vi "运维调试_五参数.vi"(11 "编号":string) -> ()   [LabVIEW 2016, in "斯坦道多参数.lvlib"]
uses:
  <vilib>/Utility/miscctls.llb/LVPointTypeDef.ctl
  <vilib>/Plasmionique/MB Master/MB_Master_Serial/MB_Master_Serial.lvclass
  <vilib>/Utility/config.llb/NI_LVConfig.lvlib
panel:
  in  "权限2":bool
  out "权限1":bool
  out "密码":dbl
  in  "密码锁":bool
  in  "蓝绿藻探头选择":u16(ring) items=["禹山", "国弘", "纳清"]
  in  "叶绿素a探头选择":u16(ring) items=["禹山", "国弘", "纳清"]
  in  "浊度探头选择":u16(ring) items=["禹山", "国弘"]
  in  "电导率探头选择":u16(ring) items=["禹山", "国弘"]
  in  "DO探头选择":u16(ring) items=["禹山", "国弘"]
  in  "pH探头选择":u16(ring) items=["禹山", "国弘"]
  in  "设置页返回":bool
  in  "蓝绿藻":bool
  in  "打开串口":bool
  in  "叶绿素a启用":bool
  in  "Temp":bool
  in  "Cond":bool
  in  "Turb":bool
  in  "DO":bool
  in  "pH":bool
  in  "VISA资源名称":refnum<visa-resource-name>
  in  "周期设置":bool
  out "当前串口":string
  out "运行状态":u16(ring) items=["空闲", "水样测试", "标样核查"]
  in  "叶绿素a校准":bool
  in  "停止":bool
  in  "标样核查":bool
  in  "水样测试":bool
  in  "open MB":bool
  in  "设置":bool
  in  "水温校准":bool
  in  "浊度校准":bool
  in  "溶解氧校准":bool
  in  "电导率校准":bool
  in  "pH校准":bool
  in  "探头校正返回":bool
  in  "探头校正":bool
  out "检测值":T1
  # "请设置串口参数"
  # "请选择要启用的参数"
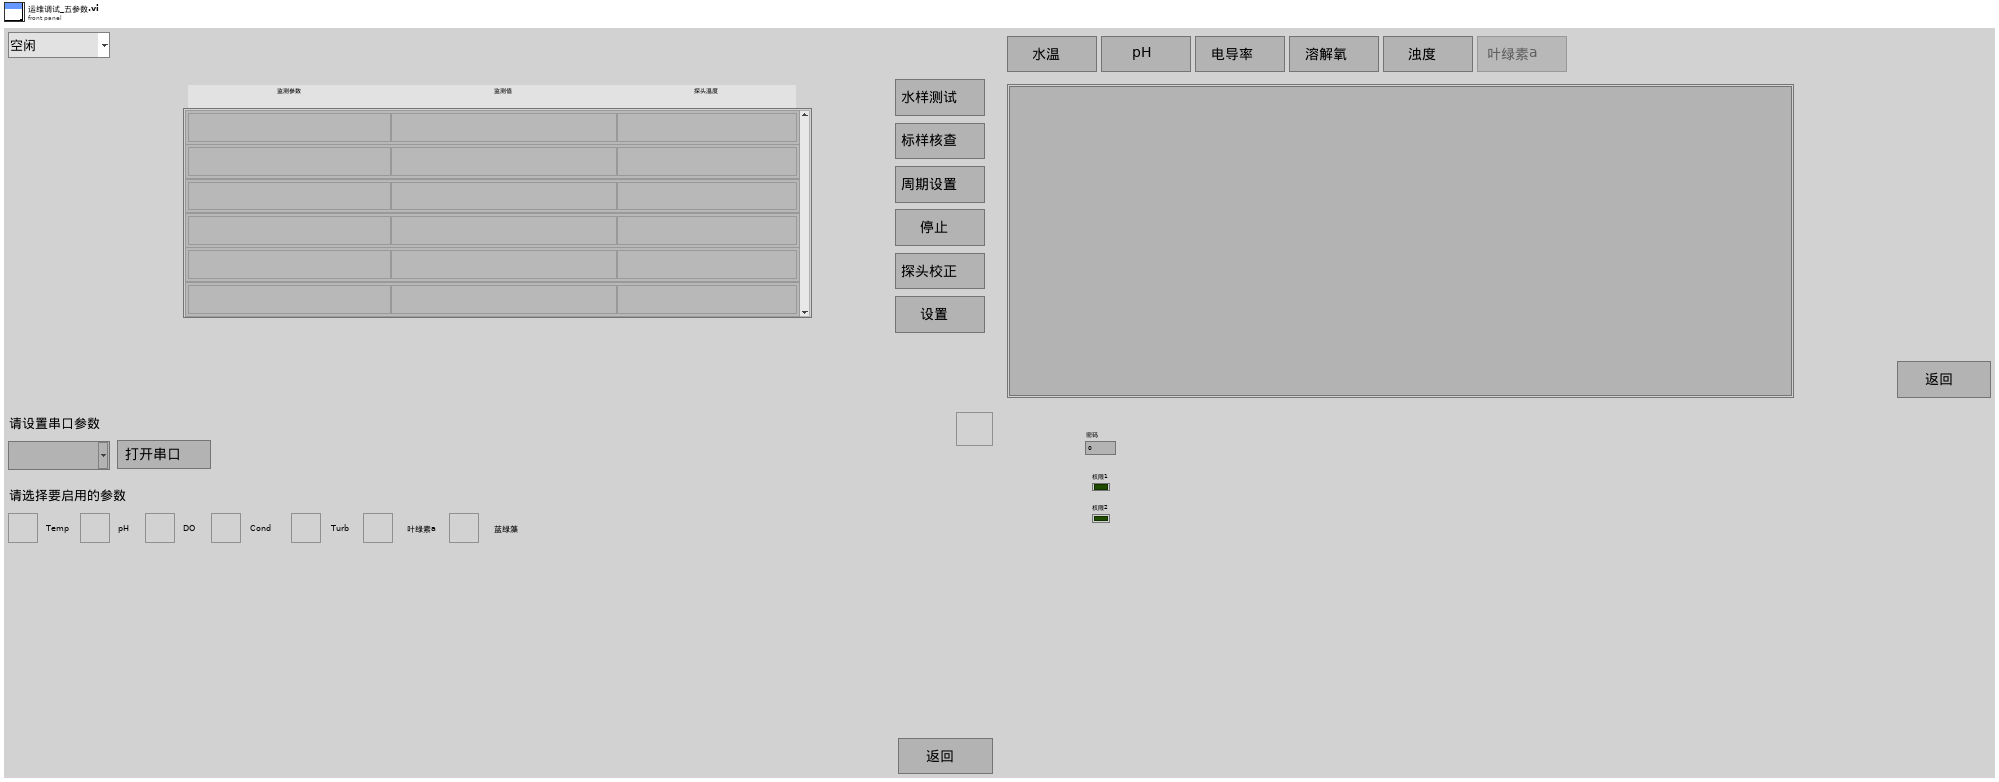
[diagram p1: front panel]
types:
  T1 = typedef "斯坦道多参数.lvlib/检测值.ctl" = cluster{"监测参数1":string, "浓度1":string, "探头温度1":string}[]
  T2 = typedef "LVPointTypeDef.ctl" = cluster{"Horizontal":i16, "Vertical":i16}
  T3 = cluster{"pH探头选择":u16, "DO探头选择":u16, "电导率探头选择":u16, "浊度探头选择":u16, "叶绿素a探头选择":u16, "蓝绿藻探头选择":u16}
  T4 = cluster{"温度测量值":sgl, "DO%":sgl, "DOmg/L":sgl, "温度偏移修正值":sgl}
  T5 = cluster{"电极状态标志":u16, "电极型号标志":u16, "溶解氧测量值":sgl, "温度测量值":sgl, "溶解氧饱和度值":sgl, "盐度补偿值":sgl, "大气压补偿值":sgl, "溶解氧偏移修正值":sgl, "温度偏移修正值":sgl, "手动温度补偿值":sgl, "溶解氧电极零点":sgl, "溶解氧电极斜率":sgl, "第1点标准值记录":sgl, "第1点信号值记录":sgl, "第1点温度值记录":sgl, "第2点标准值记录":sgl, "第2点信号值记录":sgl, "第2点温度值记录":sgl, "命令滤波设定":u16, "温度模式":enum16{"ATC", "MTC"}, "生产批次":u16, "电极序号":u16, "串口地址":u16, "串口波特率":enum16{"9600", "19200", "115200"}, "串口校验位":enum16{"NONE", "ODD", "EVEN"}, "串口停止位":enum16{"1bit", "2bit"}, "第一点标准值":sgl, "第二点标准值":sgl}
  T6 = cluster{"电极状态标志":u16, "电极型号标志":u16, "酸碱度测量值":sgl, "温度测量值":sgl, "酸碱度信号值":sgl, "温度信号值":sgl, "酸碱度偏移修正值":sgl, "温度偏移修正值":sgl, "手动温度补偿值":sgl, "酸碱度电极零点":sgl, "酸碱度电极斜率":sgl, "第1点标准值记录":sgl, "第1点信号值记录":sgl, "第1点温度值记录":sgl, "第2点标准值记录":sgl, "第2点信号值记录":sgl, "第2点温度值记录":sgl, "命令滤波设定":u16, "温度模式":enum16{"ATC", "MTC"}, "生产批次":u16, "电极序号":u16, "串口地址":u16, "串口波特率":enum16{"9600", "19200", "115200"}, "串口校验位":enum16{"NONE", "ODD", "EVEN"}, "串口停止位":enum16{"1bit", "2bit"}, "第一点标准值":sgl, "第二点标准值":sgl}
  T7 = cluster{"电极状态标志":u16, "电极型号标志":u16, "浊度测量值":sgl, "温度测量值":sgl, "浊度信号值":sgl, "浊度偏移修正值":sgl, "温度偏移修正值":sgl, "手动温度补偿值":sgl, "浊度电极零点":sgl, "浊度电极斜率":sgl, "第1点标准值记录":sgl, "第1点信号值记录":sgl, "第1点温度值记录":sgl, "第2点标准值记录":sgl, "第2点信号值记录":sgl, "第2点温度值记录":sgl, "命令滤波设定":u16, "温度模式":enum16{"ATC", "MTC"}, "生产批次":u16, "电极序号":u16, "串口地址":u16, "串口波特率":enum16{"9600", "19200", "115200"}, "串口校验位":enum16{"NONE", "ODD", "EVEN"}, "串口停止位":enum16{"1bit", "2bit"}, "第一点标准值":sgl, "第二点标准值":sgl, "第三点标准值":sgl}
  T8 = cluster{"电极状态标志":u16, "电极型号标志":u16, "电导率测量值":sgl, "温度测量值":sgl, "电导率信号值":sgl, "温度信号值":sgl, "温度补偿系数":sgl, "电导率偏移修正值":sgl, "温度偏移修正值":sgl, "手动温度补偿值":sgl, "电导率电极零点":sgl, "电导率电极斜率":sgl, "命令滤波设定":u16, "温度模式":enum16{"ATC", "MTC"}, "生产批次":u16, "电极序号":u16, "串口地址":u16, "串口波特率":enum16{"9600", "19200", "115200"}, "串口校验位":enum16{"NONE", "ODD", "EVEN"}, "串口停止位":enum16{"1bit", "2bit"}, "第一点标准值":sgl, "第二点标准值":sgl}
  T9 = enum8{"Enabled", "Disabled", "Disabled and Grayed Out"}
  T10 = cluster{"监测参数1":string, "浓度1":string, "探头温度1":string}[]
  T11 = cluster{"周期设置类型":enum16{"定点启动", "间隔启动"}, "定时功能启用":bool, "定时间隔":u32, "24H周期设置":bool[]}
  T12 = enum32{"Bad", "Idle", "Run top level", "Running"}
  T13 = typedef "LVDateTimeRec.ctl" = cluster{"秒数的小数部分":dbl, "秒":i32, "分":i32, "时":i32, "日":i32, "月":i32, "年":i32, "天数（周）":i32, "天数（年）":i32, "DST":i32}
  T14 = typedef "NI_LVConfig.lvlib/Config Data RefNum.ctl" = refnum<k1>
  T15 = cluster{"数据保存间隔":dbl, "水温标样值":dbl, "pH标样值":dbl, "溶解氧标样值":dbl, "电导率标样值":dbl, "浊度标样值":dbl}
  T16 = cluster{"baud rate (bps)":u32, "stop bits":u16, "parity":u16, "flow control":u16, "timeout":u32, "retries":i32}
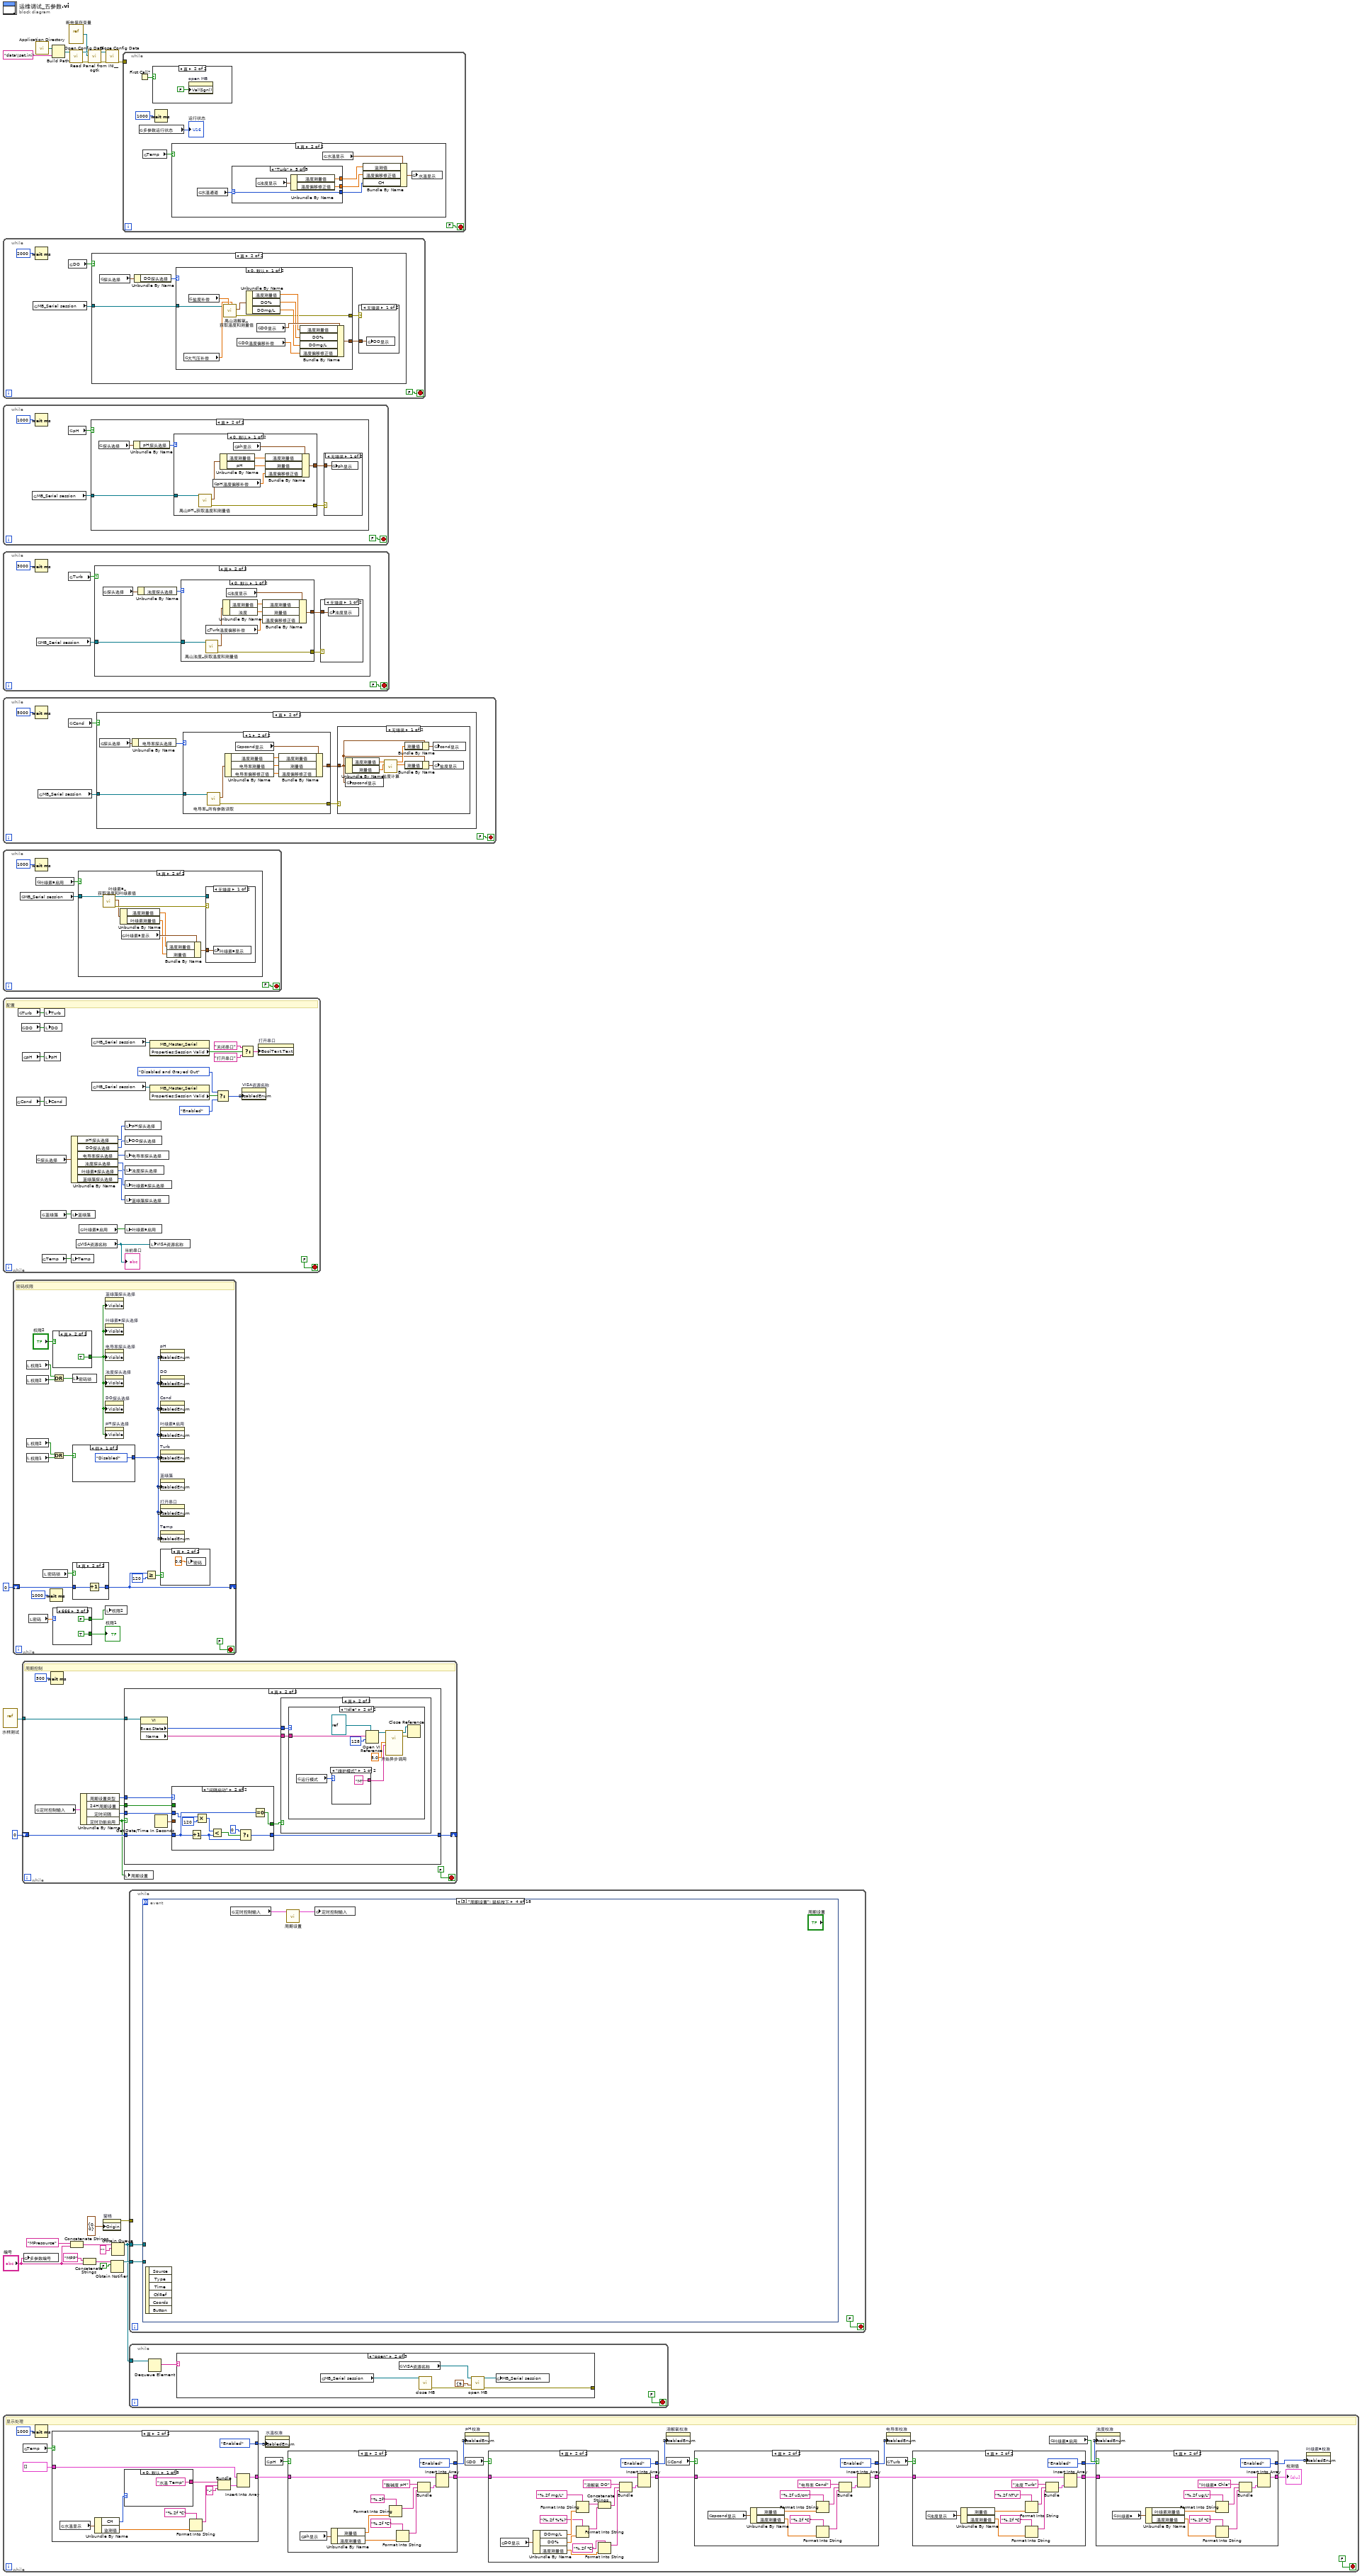
[diagram p0: block diagram]
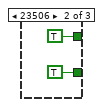
[diagram p5: hidden frame]
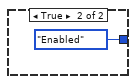
[diagram p6: hidden frame]
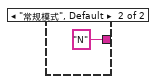
[diagram p11: hidden frame]
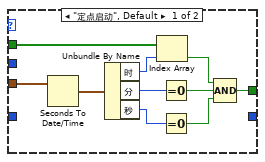
[diagram p12: hidden frame]
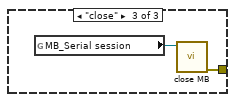
[diagram p14: hidden frame]
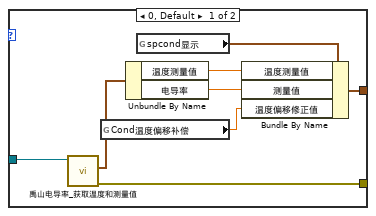
[diagram p18: hidden frame]
diagram:
  n1 = while {
    stop <- FALSE stop-if-true
    n2 = global read "多参数全局变量.vi" "MB_Serial session"() -> (w24:refnum<class "MB_Master_Serial.lvclass">)
    n3 = Wait (ms)(milliseconds to wait=u32 2000 ("等待时间（毫秒）")) -> ()  [unwired: 1 out]
    n4 = global read "断电保存变量.vi" "DO"() -> (w25:bool)
    n5 = case shown="真" w25 {
      tunnel: w24 -> [_ w30]
      frame False {
      }
      frame True {
        n6 = global read "断电保存变量.vi" "探头选择"() -> (w32:T3)
        n7 = Unbundle By Name(w32) -> ("DO探头选择"=w31:u16)
        n8 = case shown="0, 默认" w31 {
          tunnel: w30 -> [w41 w51]
          tunnel: [w39 w49] -> w29
          tunnel: [w35 w44] -> w28
          frame 0, Default {
            n9 = global read "断电保存变量.vi" "大气压补偿"() -> (w42:dbl)
            n10 = global read "断电保存变量.vi" "盐度补偿"() -> (w43:dbl)
            n11 = call "禹山溶解氧_获取温度和测量值.vi"("大气压补偿"=w42, "盐度补偿"=w43, "MB_Serial session in"=w41) -> ("error out"=w35:errorcluster, "输出值"=w33:cluster{"温度测量值":sgl, "DO%":sgl, "DOmg/L":sgl})  [unwired: 6 in, 1 out]
            n12 = global read "断电保存变量.vi" "DO温度偏移补偿"() -> (w34:dbl)
            n13 = Unbundle By Name(w33) -> ("温度测量值"=w38:sgl, "DO%"=w37:sgl, "DOmg/L"=w36:sgl)
            n14 = global read "多参数全局变量.vi" "DO显示"() -> (w40:T4)
            n15 = Bundle By Name(cluster=w40, "温度测量值"=w38, "DO%"=w37, "DOmg/L"=w36, "温度偏移修正值"=w34) -> (w39:T4)
          }
          frame 1 {
            n16 = call "DO_所有参数读取.vi"("MB_Serial session in"=w51) -> ("error out"=w44:errorcluster, "输出值"=w48:T5)  [unwired: 8 in, 1 out]
            n17 = Unbundle By Name(w48) -> ("温度测量值"=w45:sgl, "溶解氧饱和度值"=w46:sgl, "溶解氧测量值"=w47:sgl)
            n18 = global read "多参数全局变量.vi" "DO显示"() -> (w50:T4)
            n19 = Bundle By Name(cluster=w50, "温度测量值"=w45, "DO%"=w46, "DOmg/L"=w47) -> (w49:T4)
          }
        }
        n20 = case shown="无错误" w28 {
          tunnel: w29 -> [w52 _]
          frame No Error {
            n21 = global write "多参数全局变量.vi" "DO显示"(w52) -> ()
          }
          frame Error {
          }
        }
      }
    }
  }
  n22 = while {
    stop <- FALSE stop-if-true
    n23 = global read "多参数全局变量.vi" "MB_Serial session"() -> (w53:refnum<class "MB_Master_Serial.lvclass">)
    n24 = Wait (ms)(milliseconds to wait=u32 1000 ("等待时间（毫秒）")) -> ()  [unwired: 1 out]
    n25 = global read "断电保存变量.vi" "pH"() -> (w55:bool)
    n26 = case shown="真" w55 {
      tunnel: w53 -> [_ w59]
      frame False {
      }
      frame True {
        n27 = global read "断电保存变量.vi" "探头选择"() -> (w61:T3)
        n28 = Unbundle By Name(w61) -> ("pH探头选择"=w60:u16)
        n29 = case shown="0, 默认" w60 {
          tunnel: w59 -> [w69 w77]
          tunnel: [w68 w76] -> w58
          tunnel: [w66 w73] -> w57
          frame 0, Default {
            n30 = call "禹山pH_获取温度和测量值.vi"("MB_Serial session in"=w69) -> ("error out"=w68:errorcluster, "输出值"=w65:cluster{"温度测量值":sgl, "ORP":sgl, "pH":sgl})  [unwired: 8 in, 1 out]
            n31 = global read "断电保存变量.vi" "pH温度偏移补偿"() -> (w62:dbl)
            n32 = Unbundle By Name(w65) -> ("温度测量值"=w64:sgl, "pH"=w63:sgl)
            n33 = global read "多参数全局变量.vi" "ph显示"() -> (w67:cluster{"温度测量值":sgl, "测量值":sgl, "温度偏移修正值":sgl})
            n34 = Bundle By Name(cluster=w67, "温度测量值"=w64, "测量值"=w63, "温度偏移修正值"=w62) -> (w66:cluster{"温度测量值":sgl, "测量值":sgl, "温度偏移修正值":sgl})
          }
          frame 1 {
            n35 = call "pH_所有参数读取.vi"("MB_Serial session in"=w77) -> ("error out"=w76:errorcluster, "输出值"=w75:T6)  [unwired: 8 in, 1 out]
            n36 = Unbundle By Name(w75) -> ("温度测量值"=w70:sgl, "酸碱度测量值"=w71:sgl, "温度偏移修正值"=w72:sgl)
            n37 = global read "多参数全局变量.vi" "ph显示"() -> (w74:cluster{"温度测量值":sgl, "测量值":sgl, "温度偏移修正值":sgl})
            n38 = Bundle By Name(cluster=w74, "温度测量值"=w70, "测量值"=w71, "温度偏移修正值"=w72) -> (w73:cluster{"温度测量值":sgl, "测量值":sgl, "温度偏移修正值":sgl})
          }
        }
        n39 = case shown="无错误" w58 {
          tunnel: w57 -> [w78 _]
          frame No Error {
            n40 = global write "多参数全局变量.vi" "ph显示"(w78) -> ()
          }
          frame Error {
          }
        }
      }
    }
  }
  n41 = while {
    stop <- FALSE stop-if-true
    n42 = Wait (ms)(milliseconds to wait=u32 3000 ("等待时间（毫秒）")) -> ()  [unwired: 1 out]
    n43 = global read "多参数全局变量.vi" "MB_Serial session"() -> (w79:refnum<class "MB_Master_Serial.lvclass">)
    n44 = global read "断电保存变量.vi" "Turb"() -> (w81:bool)
    n45 = case shown="真" w81 {
      tunnel: w79 -> [_ w85]
      frame False {
      }
      frame True {
        n46 = global read "断电保存变量.vi" "探头选择"() -> (w87:T3)
        n47 = Unbundle By Name(w87) -> ("浊度探头选择"=w86:u16)
        n48 = case shown="0, 默认" w86 {
          tunnel: w85 -> [w95 w102]
          tunnel: [w93 w97] -> w84
          tunnel: [w92 w96] -> w83
          frame 0, Default {
            n49 = call "禹山浊度_获取温度和测量值.vi"("MB_Serial session in"=w95) -> ("error out"=w92:errorcluster, "输出值"=w91:cluster{"温度测量值":sgl, "浊度":sgl})  [unwired: 8 in, 1 out]
            n50 = global read "断电保存变量.vi" "Turb温度偏移补偿"() -> (w88:dbl)
            n51 = Unbundle By Name(w91) -> ("温度测量值"=w90:sgl, "浊度"=w89:sgl)
            n52 = global read "多参数全局变量.vi" "浊度显示"() -> (w94:cluster{"温度测量值":sgl, "测量值":sgl, "温度偏移修正值":sgl})
            n53 = Bundle By Name(cluster=w94, "温度测量值"=w90, "测量值"=w89, "温度偏移修正值"=w88) -> (w93:cluster{"温度测量值":sgl, "测量值":sgl, "温度偏移修正值":sgl})
          }
          frame 1 {
            n54 = call "浊度_所有参数读取.vi"("MB_Serial session in"=w102) -> ("error out"=w96:errorcluster, "输出值"=w101:T7)  [unwired: 8 in, 1 out]
            n55 = Unbundle By Name(w101) -> ("温度测量值"=w99:sgl, "浊度测量值"=w98:sgl)
            n56 = global read "多参数全局变量.vi" "浊度显示"() -> (w100:cluster{"温度测量值":sgl, "测量值":sgl, "温度偏移修正值":sgl})
            n57 = Bundle By Name(cluster=w100, "温度测量值"=w99, "测量值"=w98) -> (w97:cluster{"温度测量值":sgl, "测量值":sgl, "温度偏移修正值":sgl})
          }
        }
        n58 = case shown="无错误" w83 {
          tunnel: w84 -> [w103 _]
          frame No Error {
            n59 = global write "多参数全局变量.vi" "浊度显示"(w103) -> ()
          }
          frame Error {
          }
        }
      }
    }
  }
  n60 = while {
    stop <- FALSE stop-if-true
    n61 = Wait (ms)(milliseconds to wait=u32 5000 ("等待时间（毫秒）")) -> ()  [unwired: 1 out]
    n62 = global read "多参数全局变量.vi" "MB_Serial session"() -> (w104:refnum<class "MB_Master_Serial.lvclass">)
    n63 = global read "断电保存变量.vi" "Cond"() -> (w106:bool)
    n64 = case shown="真" w106 {
      tunnel: w104 -> [_ w110]
      frame False {
      }
      frame True {
        n65 = global read "断电保存变量.vi" "探头选择"() -> (w112:T3)
        n66 = Unbundle By Name(w112) -> ("电导率探头选择"=w111:u16)
        n67 = case shown="1" w111 {
          tunnel: w110 -> [w120 w128]
          tunnel: [w114 w126] -> w109
          tunnel: [w119 w125] -> w108
          frame 0, Default {
            n68 = call "禹山电导率_获取温度和测量值.vi"("MB_Serial session in"=w120) -> ("error out"=w119:errorcluster, "输出值"=w117:cluster{"温度测量值":sgl, "电导率":sgl, "错误标志":u16})  [unwired: 8 in, 1 out]
            n69 = global read "断电保存变量.vi" "Cond温度偏移补偿"() -> (w113:dbl)
            n70 = Unbundle By Name(w117) -> ("温度测量值"=w116:sgl, "电导率"=w115:sgl)
            n71 = global read "多参数全局变量.vi" "spcond显示"() -> (w118:cluster{"温度测量值":sgl, "测量值":sgl, "温度偏移修正值":sgl})
            n72 = Bundle By Name(cluster=w118, "温度测量值"=w116, "测量值"=w115, "温度偏移修正值"=w113) -> (w114:cluster{"温度测量值":sgl, "测量值":sgl, "温度偏移修正值":sgl})
          }
          frame 1 {
            n73 = call "电导率_所有参数读取.vi"("MB_Serial session in"=w128) -> ("error out"=w125:errorcluster, "输出值"=w124:T8)  [unwired: 8 in, 1 out]
            n74 = Unbundle By Name(w124) -> ("温度测量值"=w123:sgl, "电导率测量值"=w122:sgl, "电导率偏移修正值"=w121:sgl)
            n75 = global read "多参数全局变量.vi" "spcond显示"() -> (w127:cluster{"温度测量值":sgl, "测量值":sgl, "温度偏移修正值":sgl})
            n76 = Bundle By Name(cluster=w127, "温度测量值"=w123, "测量值"=w122, "温度偏移修正值"=w121) -> (w126:cluster{"温度测量值":sgl, "测量值":sgl, "温度偏移修正值":sgl})
          }
        }
        n77 = case shown="无错误" w108 {
          tunnel: w109 -> [w130 _]
          frame No Error {
            n78 = Unbundle By Name(w130) -> ("温度测量值"=w135:sgl, "测量值"=w134:sgl)
            n79 = global write "多参数全局变量.vi" "spcond显示"(w130) -> ()
            n80 = call "盐度计算.vi"("spCond"=w134, "Temp"=w135) -> ("saltresult"=w129:dbl, "cond"=w133:dbl)  [unwired: 8 in]
            n81 = Bundle By Name(cluster=w130, "测量值"=w133) -> (w132:cluster{"温度测量值":sgl, "测量值":sgl, "温度偏移修正值":sgl})
            n82 = Bundle By Name(cluster=w130, "测量值"=w129) -> (w131:cluster{"温度测量值":sgl, "测量值":sgl, "温度偏移修正值":sgl})
            n83 = global write "多参数全局变量.vi" "cond显示"(w132) -> ()
            n84 = global write "多参数全局变量.vi" "盐度显示"(w131) -> ()
          }
          frame Error {
          }
        }
      }
    }
  }
  n85 = while {
    stop <- FALSE stop-if-true
    n86 = global read "多参数全局变量.vi" "MB_Serial session"() -> (w136:refnum<class "MB_Master_Serial.lvclass">)
    n87 = Wait (ms)(milliseconds to wait=u32 1000 ("等待时间（毫秒）")) -> ()  [unwired: 1 out]
    n88 = global read "断电保存变量.vi" "叶绿素a启用"() -> (w138:bool)
    n89 = case shown="真" w138 {
      tunnel: w136 -> [_ w145]
      frame False {
      }
      frame True {
        n90 = call "叶绿素a_获取温度和叶绿素值.vi"("MB_Serial session in"=w145) -> ("error out"=w147:errorcluster, "输出值"=w142:cluster{"温度测量值":sgl, "叶绿素测量值":sgl, "错误标志":u16}, "MB_Serial session out"=w146:refnum<class "MB_Master_Serial.lvclass">)  [unwired: 8 in]
        n91 = Unbundle By Name(w142) -> ("温度测量值"=w140:sgl, "叶绿素测量值"=w141:sgl)
        n92 = global read "多参数全局变量.vi" "叶绿素a显示"() -> (w144:cluster{"温度测量值":sgl, "测量值":sgl, "温度偏移修正值":sgl})
        n93 = Bundle By Name(cluster=w144, "温度测量值"=w140, "测量值"=w141) -> (w143:cluster{"温度测量值":sgl, "测量值":sgl, "温度偏移修正值":sgl})
        n94 = case shown="无错误" w147 {
          tunnel: w146 -> [_ _]
          tunnel: w143 -> [w148 _]
          frame No Error {
            n95 = global write "多参数全局变量.vi" "叶绿素a显示"(w148) -> ()
          }
          frame Error {
          }
        }
      }
    }
  }
  n96 = while {
    stop <- FALSE stop-if-true
    # "配置"
    n97 = global read "断电保存变量.vi" "Cond"() -> (w170:bool)
    n98 = global read "断电保存变量.vi" "Turb"() -> (w169:bool)
    n99 = global read "断电保存变量.vi" "DO"() -> (w171:bool)
    n100 = global read "断电保存变量.vi" "pH"() -> (w172:bool)
    n101 = global read "断电保存变量.vi" "探头选择"() -> (w155:T3)
    n102 = global read "断电保存变量.vi" "蓝绿藻"() -> (w167:bool)
    n103 = global read "断电保存变量.vi" "Temp"() -> (w173:bool)
    n104 = local write "Turb"(w169) -> ()
    n105 = local write "DO"(w171) -> ()
    n106 = local write "pH"(w172) -> ()
    n107 = local write "Cond"(w170) -> ()
    n108 = Unbundle By Name(w155) -> ("pH探头选择"=w154:u16, "DO探头选择"=w153:u16, "电导率探头选择"=w152:u16, "浊度探头选择"=w151:u16, "叶绿素a探头选择"=w150:u16, "蓝绿藻探头选择"=w149:u16)
    n109 = local write "蓝绿藻"(w167) -> ()
    n110 = local write "Temp"(w173) -> ()
    n111 = global read "断电保存变量.vi" "VISA资源名称"() -> (w156:refnum<visa-resource-name>)
    "当前串口" <- w156
    n112 = global read "断电保存变量.vi" "叶绿素a启用"() -> (w168:bool)
    n113 = global read "多参数全局变量.vi" "MB_Serial session"() -> (w161:refnum<class "MB_Master_Serial.lvclass">)
    n114 = global read "多参数全局变量.vi" "MB_Serial session"() -> (w166:refnum<class "MB_Master_Serial.lvclass">)
    n115 = local write "pH探头选择"(w154) -> ()
    n116 = local write "DO探头选择"(w153) -> ()
    n117 = local write "电导率探头选择"(w152) -> ()
    n118 = local write "浊度探头选择"(w151) -> ()
    n119 = local write "叶绿素a探头选择"(w150) -> ()
    n120 = local write "蓝绿藻探头选择"(w149) -> ()
    n121 = local write "叶绿素a启用"(w168) -> ()
    n122 = property class="MB_Master_Serial"(reference=w161) -> ("Properties:Session Valid"=w160:bool)  [unwired: 1 in, 2 out]
    n123 = property class="MB_Master_Serial"(reference=w166) -> ("Properties:Session Valid"=w165:bool)  [unwired: 1 in, 2 out]
    n124 = local write "VISA资源名称"(w156) -> ()
    n125 = Select(t=T9."Disabled and Grayed Out" ("禁用"), s=w165, f=T9."Enabled") -> (s? t:f=w163:T9)
    n126 = Select(t="关闭串口" ("布尔文本.文本"), s=w160, f="打开串口" ("布尔文本.文本")) -> (s? t:f=w157:string)
    n127 = property on="VISA资源名称" class="VISAName"("DisabledEnum"=w163) -> ()  [unwired: 2 in, 2 out]
    n128 = property on="打开串口" class="Bool"("BoolText.Text"=w157) -> ()  [unwired: 2 in, 2 out]
  }
  n129 = vi-ref "水样测试.vi"() -> (w2:refnum<vi>)
  n130 = while {
    stop <- FALSE stop-if-true
    # "显示处理"
    n131 = global read "断电保存变量.vi" "Temp"() -> (w193:bool)
    n132 = Wait (ms)(milliseconds to wait=u32 1000 ("等待时间（毫秒）")) -> ()  [unwired: 1 out]
    n133 = case shown="真" w193 {
      tunnel: [w271 w276] -> w190
      tunnel: T10 [] ("数组") -> [w271 w277]
      tunnel: [T9."Disabled and Grayed Out" ("禁用") T9."Enabled" ("禁用")] -> w175
      frame False {
      }
      frame True {
        n134 = global read "多参数全局变量.vi" "水温显示"() -> (w274:cluster{"CH":u16, "监测值":dbl, "温度偏移修正值":sgl})
        n135 = Unbundle By Name(w274) -> ("CH"=w273:u16, "监测值"=w272:dbl)
        n136 = case shown="0, 默认" w273 {
          tunnel: ["水温 Temp" ("监测参数1") "水温 Temp (pH)" ("监测参数1") "水温 Temp (Cond)" ("监测参数1") "水温 Temp (DO)" ("监测参数1") "水温 Temp (Turb)" ("监测参数1")] -> w281
          frame 0, Default {
          }
          frame 1 {
          }
          frame 2 {
          }
          frame 3 {
          }
          frame 4 {
          }
        }
        n137 = Format Into String(format string="%.2f ℃" ("格式字符串"), w272) -> (resulting string=w280:string)  [unwired: 2 in, 1 out]
        n138 = Bundle("监测参数1"=w281, w280, "探头温度1"="-") -> (w278:cluster{"监测参数1":string, string, "探头温度1":string})  [unwired: 1 in]
        n139 = Insert Into Array(array=w277, new element=w278) -> (w276:T10)  [unwired: 1 in]
      }
    }
    n140 = property on="水温校准" class="Bool"("DisabledEnum"=w175) -> ()  [unwired: 2 in, 2 out]
    n141 = global read "断电保存变量.vi" "pH"() -> (w191:bool)
    n142 = case shown="真" w191 {
      tunnel: [w257 w260] -> w188
      tunnel: w190 -> [w257 w262]
      tunnel: [T9."Disabled and Grayed Out" ("禁用") T9."Enabled" ("禁用")] -> w180
      frame False {
      }
      frame True {
        n143 = global read "多参数全局变量.vi" "ph显示"() -> (w258:cluster{"温度测量值":sgl, "测量值":sgl, "温度偏移修正值":sgl})
        n144 = Unbundle By Name(w258) -> ("测量值"=w269:sgl, "温度测量值"=w267:sgl)
        n145 = Format Into String(format string="%.2f" ("格式字符串"), w269) -> (resulting string=w263:string)  [unwired: 2 in, 1 out]
        n146 = Format Into String(format string="%.2f ℃" ("格式字符串"), w267) -> (resulting string=w265:string)  [unwired: 2 in, 1 out]
        n147 = Bundle("监测参数2"="酸碱度 pH", w263, w265) -> (w261:cluster{"监测参数2":string, string, string})  [unwired: 1 in]
        n148 = Insert Into Array(array=w262, new element=w261) -> (w260:T10)  [unwired: 1 in]
      }
    }
    n149 = property on="pH校准" class="Bool"("DisabledEnum"=w180) -> ()  [unwired: 2 in, 2 out]
    n150 = global read "断电保存变量.vi" "DO"() -> (w189:bool)
    n151 = case shown="真" w189 {
      tunnel: [w239 w242] -> w185
      tunnel: w188 -> [w239 w243]
      tunnel: [T9."Disabled and Grayed Out" ("禁用") T9."Enabled" ("禁用")] -> w179
      frame False {
      }
      frame True {
        n152 = global read "多参数全局变量.vi" "DO显示"() -> (w240:T4)
        n153 = Unbundle By Name(w240) -> ("DOmg/L"=w252:sgl, "DO%"=w250:sgl, "温度测量值"=w254:sgl)
        n154 = Format Into String(format string="%.2f mg/L" ("格式字符串"), w252) -> (resulting string=w249:string)  [unwired: 2 in, 1 out]
        n155 = Format Into String(format string="(%.2f %%)" ("格式字符串"), w250) -> (resulting string=w248:string)  [unwired: 2 in, 1 out]
        n156 = Concatenate Strings(w249, w248) -> (w247:string)
        n157 = Format Into String(format string="%.2f ℃" ("格式字符串"), w254) -> (resulting string=w245:string)  [unwired: 2 in, 1 out]
        n158 = Bundle("监测参数2"="溶解氧 DO", w247, w245) -> (w244:cluster{"监测参数2":string, string, string})  [unwired: 1 in]
        n159 = Insert Into Array(array=w243, new element=w244) -> (w242:T10)  [unwired: 1 in]
      }
    }
    n160 = property on="溶解氧校准" class="Bool"("DisabledEnum"=w179) -> ()  [unwired: 2 in, 2 out]
    n161 = global read "断电保存变量.vi" "Cond"() -> (w187:bool)
    n162 = case shown="真" w187 {
      tunnel: w185 -> [w225 w232]
      tunnel: [w225 w230] -> w184
      tunnel: [T9."Disabled and Grayed Out" ("禁用") T9."Enabled" ("禁用")] -> w178
      frame False {
      }
      frame True {
        n163 = global read "多参数全局变量.vi" "spcond显示"() -> (w228:cluster{"温度测量值":sgl, "测量值":sgl, "温度偏移修正值":sgl})
        n164 = Unbundle By Name(w228) -> ("测量值"=w227:sgl, "温度测量值"=w226:sgl)
        n165 = Format Into String(format string="%.2f uS/cm" ("格式字符串"), w227) -> (resulting string=w233:string)  [unwired: 2 in, 1 out]
        n166 = Format Into String(format string="%.2f ℃" ("格式字符串"), w226) -> (resulting string=w234:string)  [unwired: 2 in, 1 out]
        n167 = Bundle("监测参数2"="电导率 Cond", w233, w234) -> (w231:cluster{"监测参数2":string, string, string})  [unwired: 1 in]
        n168 = Insert Into Array(array=w232, new element=w231) -> (w230:T10)  [unwired: 1 in]
      }
    }
    n169 = property on="电导率校准" class="Bool"("DisabledEnum"=w178) -> ()  [unwired: 2 in, 2 out]
    n170 = global read "断电保存变量.vi" "Turb"() -> (w186:bool)
    n171 = case shown="真" w186 {
      tunnel: w184 -> [w211 w218]
      tunnel: [w211 w216] -> w183
      tunnel: [T9."Disabled and Grayed Out" ("禁用") T9."Enabled" ("禁用")] -> w177
      frame False {
      }
      frame True {
        n172 = global read "多参数全局变量.vi" "浊度显示"() -> (w214:cluster{"温度测量值":sgl, "测量值":sgl, "温度偏移修正值":sgl})
        n173 = Unbundle By Name(w214) -> ("测量值"=w213:sgl, "温度测量值"=w212:sgl)
        n174 = Format Into String(format string="%.2f NTU" ("格式字符串"), w213) -> (resulting string=w220:string)  [unwired: 2 in, 1 out]
        n175 = Format Into String(format string="%.2f ℃" ("格式字符串"), w212) -> (resulting string=w221:string)  [unwired: 2 in, 1 out]
        n176 = Bundle("监测参数2"="浊度 Turb", w220, w221) -> (w217:cluster{"监测参数2":string, string, string})  [unwired: 1 in]
        n177 = Insert Into Array(array=w218, new element=w217) -> (w216:T10)  [unwired: 1 in]
      }
    }
    n178 = global read "断电保存变量.vi" "叶绿素a启用"() -> (w181:bool)
    n179 = property on="浊度校准" class="Bool"("DisabledEnum"=w177) -> ()  [unwired: 2 in, 2 out]
    n180 = case shown="真" w181 {
      tunnel: w183 -> [w197 w204]
      tunnel: [w197 w202] -> w182
      tunnel: [T9."Disabled and Grayed Out" ("禁用") T9."Enabled" ("禁用")] -> w176
      frame False {
      }
      frame True {
        n181 = global read "禹山过程全局变量.vi" "叶绿素a"() -> (w201:cluster{"温度测量值":sgl, "叶绿素测量值":sgl, "错误标志":u16})
        n182 = Unbundle By Name(w201) -> ("叶绿素测量值"=w200:sgl, "温度测量值"=w199:sgl)
        n183 = Format Into String(format string="%.2f ug/L" ("格式字符串"), w200) -> (resulting string=w206:string)  [unwired: 2 in, 1 out]
        n184 = Format Into String(format string="%.2f ℃" ("格式字符串"), w199) -> (resulting string=w207:string)  [unwired: 2 in, 1 out]
        n185 = Bundle("监测参数2"="叶绿素a Chla", w206, w207) -> (w203:cluster{"监测参数2":string, string, string})  [unwired: 1 in]
        n186 = Insert Into Array(array=w204, new element=w203) -> (w202:T10)  [unwired: 1 in]
      }
    }
    "检测值" <- w182
    n187 = property on="叶绿素a校准" class="Bool"("DisabledEnum"=w176) -> ()  [unwired: 2 in, 2 out]
  }
  n188 = while {
    shift-right: [w290] -> _
    shift-left: u32 0 ("等待时间（毫秒）") -> [w291]
    stop <- FALSE stop-if-true
    # "密码权限"
    n189 = local read "权限1"() -> (w297:bool)
    n190 = local read "权限2"() -> (w298:bool)
    n191 = local read "权限2"() -> (w295:bool)
    n192 = local read "权限1"() -> (w303:bool)
    n193 = local read "密码"() -> (w301:dbl)
    n194 = local read "密码锁"() -> (w292:bool)
    n195 = Wait (ms)(milliseconds to wait=u32 1000 ("等待时间（毫秒）")) -> ()  [unwired: 1 out]
    n196 = Or(x=w297, y=w298) -> (x .or. y?=w294:bool)
    n197 = Or(x=w295, y=w303) -> (x .or. y?=w296:bool)
    n198 = case shown="真" "权限2" {
      tunnel: [_ TRUE ("可见")] -> w305
      frame False {
      }
      frame True {
      }
    }
    n199 = case shown="666" w301 {
      tunnel: [_ TRUE ("可见") FALSE ("可见")] -> w300
      tunnel: [_ TRUE ("可见") TRUE ("可见")] -> w299
      frame 0, Default {
      }
      frame 23506 {
      }
      frame 666 {
      }
    }
    "权限1" <- w299
    n200 = local write "密码锁"(w294) -> ()
    n201 = case shown="假" w296 {
      tunnel: [T9."Disabled" ("禁用") T9."Enabled" ("禁用")] -> w293
      frame False {
      }
      frame True {
      }
    }
    n202 = case shown="真" w292 {
      tunnel: w291 -> [_ w309]
      tunnel: [_ w308] -> w290
      frame False {
      }
      frame True {
        n203 = Increment(x=w309) -> (x+1=w308:u32)
      }
    }
    n204 = property on="蓝绿藻探头选择" class="Ring (严格)"("Visible"=w305) -> ()  [unwired: 2 in, 2 out]
    n205 = property on="叶绿素a探头选择" class="Ring (严格)"("Visible"=w305) -> ()  [unwired: 2 in, 2 out]
    n206 = property on="电导率探头选择" class="Ring (严格)"("Visible"=w305) -> ()  [unwired: 2 in, 2 out]
    n207 = property on="浊度探头选择" class="Ring (严格)"("Visible"=w305) -> ()  [unwired: 2 in, 2 out]
    n208 = property on="DO探头选择" class="Ring (严格)"("Visible"=w305) -> ()  [unwired: 2 in, 2 out]
    n209 = property on="pH探头选择" class="Ring (严格)"("Visible"=w305) -> ()  [unwired: 2 in, 2 out]
    n210 = local write "权限2"(w300) -> ()
    n211 = Greater Or Equal?(x=w290, y=u32 120) -> (x >= y?=w288:bool)
    n212 = property on="pH" class="Bool (严格)"("DisabledEnum"=w293) -> ()  [unwired: 2 in, 2 out]
    n213 = property on="DO" class="Bool (严格)"("DisabledEnum"=w293) -> ()  [unwired: 2 in, 2 out]
    n214 = property on="Cond" class="Bool (严格)"("DisabledEnum"=w293) -> ()  [unwired: 2 in, 2 out]
    n215 = property on="叶绿素a启用" class="Bool (严格)"("DisabledEnum"=w293) -> ()  [unwired: 2 in, 2 out]
    n216 = property on="Turb" class="Bool (严格)"("DisabledEnum"=w293) -> ()  [unwired: 2 in, 2 out]
    n217 = property on="蓝绿藻" class="Bool (严格)"("DisabledEnum"=w293) -> ()  [unwired: 2 in, 2 out]
    n218 = property on="打开串口" class="Bool"("DisabledEnum"=w293) -> ()  [unwired: 2 in, 2 out]
    n219 = property on="Temp" class="Bool (严格)"("DisabledEnum"=w293) -> ()  [unwired: 2 in, 2 out]
    n220 = case shown="真" w288 {
      frame False {
      }
      frame True {
        n221 = local write "密码"(0.0 ("密码")) -> ()
      }
    }
  }
  n222 = while {
    tunnel: w2 -> [w319]
    shift-right: [w318] -> _
    shift-left: u32 0 ("等待时间（毫秒）") -> [w320]
    stop <- FALSE stop-if-true
    # "周期控制"
    n223 = global read "断电保存变量.vi" "定时控制输入"() -> (w322:T11)
    n224 = Wait (ms)(milliseconds to wait=u32 500 ("等待时间（毫秒）")) -> ()  [unwired: 1 out]
    n225 = Unbundle By Name(w322) -> ("周期设置类型"=w324:enum16{"定点启动", "间隔启动"}, "24H周期设置"=w323:bool[], "定时间隔"=w321:u32, "定时功能启用"=w317:bool)
    n226 = case shown="真" w317 {
      tunnel: w324 -> [_ w335]
      tunnel: w323 -> [_ w334]
      tunnel: w321 -> [_ w332]
      tunnel: w320 -> [_ w328]
      tunnel: w319 -> [_ w331]
      tunnel: [_ w327] -> w318
      frame False {
      }
      frame True {
        n227 = property class="VI"(reference=w331) -> ("Exec.State"=w329:T12, "Name"=w330:string)  [unwired: 1 in, 2 out]
        n228 = Get Date/Time In Seconds() -> (seconds since 1Jan1904=w336:timestamp)
        n229 = case shown="\"间隔启动\"" w335 {
          tunnel: w336 -> [w359 _]
          tunnel: w334 -> [w356 _]
          tunnel: [w350 w367] -> w333
          tunnel: w332 -> [_ w366]
          tunnel: w328 -> [_ w368]
          tunnel: [_ w362] -> w327
          frame "定点启动", Default {
            n230 = Seconds To Date/Time(time stamp (now)=w359) -> (date time rec=w358:T13)  [unwired: 1 in]
            n231 = Unbundle By Name(w358) -> ("时"=w357:i32, "分"=w355:i32, "秒"=w354:i32)
            n232 = Index Array(array=w356, index=w357) -> (element=w353:bool)
            n233 = Equal To 0?(x=w355) -> (x = 0?=w352:bool)
            n234 = Equal To 0?(x=w354) -> (x = 0?=w351:bool)
            n235 = Compound Arithmetic op=AND ("复合运算")(w353, w352, w351) -> (w350:bool)
          }
          frame "间隔启动" {
            n236 = Increment(x=w368) -> (x+1=w361:u32)
            n237 = Multiply(x=w366, y=u32 120) -> (x*y=w360:u32)
            n238 = Less?(x=w360, y=w361) -> (x < y?=w364:bool)
            n239 = Select(t=u32 0 ("y"), s=w364, f=w361) -> (s? t:f=w362:u32)
            n240 = Equal To 0?(x=w368) -> (x = 0?=w367:bool)
          }
        }
        n241 = case shown="真" w333 {
          tunnel: w329 -> [_ w338]
          tunnel: w330 -> [_ w337]
          frame False {
          }
          frame True {
            n242 = case shown="\"Idle\"" w338 {
              tunnel: w337 -> [_ w344]
              frame "Bad", Default {
              }
              frame "Idle" {
                n243 = global read "多参数全局变量.vi" "运行模式"() -> (w340:enum16{"维护模式", "常规模式", "应急模式", "质控模式"})
                n244 = case shown="\"维护模式\"" w340 {
                  tunnel: ["M" ("数据标记表") "N" ("数据标记表")] -> w339
                  frame "维护模式" {
                  }
                  frame "常规模式", Default {
                  }
                }
                n245 = Open VI Reference(type specifier VI Refnum (for type only)=refnum<vi> refnum, vi path=w344, options=128 ("选项")) -> (vi reference=w345:refnum<vi>)  [unwired: 3 in, 1 out]
                n246 = call-by-ref "开始异步调用"(reference=w345, "数据标记表"=w339, "水样测试时间"=5.0) -> (reference out=w346:refnum<vi>, error out=w347:errorcluster)  [unwired: 11 in]
                n247 = Close Reference(reference=w346, error in (no error)=w347) -> ()  [unwired: 1 out]
              }
            }
          }
        }
      }
    }
    n248 = local write "周期设置"(w317) -> ()
  }
  n249 = global write "多参数全局变量.vi" "多参数编号"("编号") -> ()
  n250 = call <vilib>:"Application Directory.vi"() -> ("Application Directory"=w17:path)
  n251 = Build Path(base path=w17, name or relative path="data\\set.ini" ("名称或相对路径")) -> (appended path=w16:path)
  n252 = vi-ref "断电保存变量.vi"() -> (w14:refnum<vi>)
  n253 = call <vilib>:"Open Config Data.vi"("configuration file path"=w16) -> ("error out"=w20:errorcluster, "refnum"=w21:T14)  [unwired: 8 in, 1 out]
  n254 = Concatenate Strings("MPresource" ("名称（未命名）"), "编号") -> (w5:string)
  n255 = Concatenate Strings("MPP" ("名称（未命名）"), "编号") -> (w6:string)
  n256 = call <userlib>:"Read Panel from INI__ogtk.vi"("error in (no error)"=w20, "VI ref"=w14, "refnum"=w21) -> ("error out"=w18:errorcluster, "refnum out"=w19:T14)  [unwired: 7 in]
  n257 = property on="窗格" class="Pane"("Origin"=T2 {"Horizontal"=0, "Vertical"=0} ("原点")) -> (error out=w23:errorcluster)  [unwired: 2 in, 1 out]
  n258 = call <vilib>:"Close Config Data.vi"("error in (no error)"=w18, "refnum"=w19) -> ("error out"=w13:errorcluster)  [unwired: 8 in, 1 out]
  n259 = Obtain Notifier(name (unnamed)=w6, notification data type=FALSE) -> (notifier out=w10:refnum<notifier>)  [unwired: 2 in, 2 out]
  n260 = Obtain Queue(name (unnamed)=w5, element data type="" ("名称（未命名）")) -> (queue out=w7:refnum<queue>)  [unwired: 3 in, 2 out]
  n261 = while {
    tunnel: w13 -> [_]
    stop <- FALSE stop-if-true
    n262 = First Call?() -> (First Call?: T/F=w371:bool)
    n263 = global read "多参数全局变量.vi" "多参数运行状态"() -> (→"运行状态":u16)
    n264 = global read "断电保存变量.vi" "Temp"() -> (w370:bool)
    n265 = case shown="真" w371 {
      frame False {
      }
      frame True {
        n266 = property on="open MB" class="Bool (严格)"("Val(Sgnl)"=FALSE ("值(信号)")) -> ()  [unwired: 2 in, 2 out]
      }
    }
    n267 = Wait (ms)(milliseconds to wait=u32 1000 ("等待时间（毫秒）")) -> ()  [unwired: 1 out]
    n268 = case shown="真" w370 {
      frame False {
      }
      frame True {
        n269 = global read "断电保存变量.vi" "水温通道"() -> (w379:enum16{"NULL", "pH", "Cond", "DO", "Turb"})
        n270 = case shown="\"Turb\"" w379 {
          selector: w379 -> [w380 w384 w388 w392 w396]
          tunnel: [w380 w384 w388 w392 w396] -> w378
          tunnel: [_ w382 w385 w389 w393] -> w377
          tunnel: [_ w383 w386 w390 w394] -> w376
          frame "NULL", Default {
          }
          frame "pH" {
            n271 = global read "多参数全局变量.vi" "ph显示"() -> (w381:cluster{"温度测量值":sgl, "测量值":sgl, "温度偏移修正值":sgl})
            n272 = Unbundle By Name(w381) -> ("温度测量值"=w383:sgl, "温度偏移修正值"=w382:sgl)
          }
          frame "Cond" {
            n273 = global read "多参数全局变量.vi" "spcond显示"() -> (w387:cluster{"温度测量值":sgl, "测量值":sgl, "温度偏移修正值":sgl})
            n274 = Unbundle By Name(w387) -> ("温度测量值"=w386:sgl, "温度偏移修正值"=w385:sgl)
          }
          frame "DO" {
            n275 = global read "多参数全局变量.vi" "DO显示"() -> (w391:T4)
            n276 = Unbundle By Name(w391) -> ("温度测量值"=w390:sgl, "温度偏移修正值"=w389:sgl)
          }
          frame "Turb" {
            n277 = global read "多参数全局变量.vi" "浊度显示"() -> (w395:cluster{"温度测量值":sgl, "测量值":sgl, "温度偏移修正值":sgl})
            n278 = Unbundle By Name(w395) -> ("温度测量值"=w394:sgl, "温度偏移修正值"=w393:sgl)
          }
        }
        n279 = global read "多参数全局变量.vi" "水温显示"() -> (w374:cluster{"CH":u16, "监测值":dbl, "温度偏移修正值":sgl})
        n280 = Bundle By Name(cluster=w374, "监测值"=w376, "温度偏移修正值"=w377, "CH"=w378) -> (w375:cluster{"CH":u16, "监测值":dbl, "温度偏移修正值":sgl})
        n281 = global write "多参数全局变量.vi" "水温显示"(w375) -> ()
      }
    }
  }
  n282 = while {
    tunnel: w23 -> [_]
    tunnel: w10 -> [w399]
    tunnel: w7 -> [w398]
    stop <- FALSE stop-if-true
    n283 = event shown="[3] \"周期设置\": 鼠标按下" {
      selector: _ -> [_ _ _ _ _ _ _ _ _ _ _ _ _ _ _ _ _ _]
      dyn-events: _ -> [_ _ _ _ _ _ _ _ _ _ _ _ _ _ _ _ _ _]
      timeout: _ -> [_ _ _ _ _ _ _ _ _ _ _ _ _ _ _ _ _ _]
      tunnel: w399 -> [_ _ _ _ _ _ w440 _ _ _ _ _ _ _ _ _ _ _]
      tunnel: w398 -> [_ _ _ _ _ _ _ w443 _ _ w475 _ _ _ _ _ _ _]
      event Timeout {
        n284 = event-data() -> ()  [unwired: 1 in, 3 out]
      }
      event "VISA资源名称", "pH", "DO", "Turb", "Cond", "Temp", "叶绿素a启用", "打开串口", "蓝绿藻": Mouse Down {
        n285 = event-data() -> ()  [unwired: 1 in, 6 out]
        n286 = local read "密码锁"() -> (w401:bool)
        n287 = case shown="假" w401 {
          frame False {
            n288 = One Button Dialog(message="当前操作权限不足,请提升权限!!!" ("消息")) -> ()  [unwired: 1 in, 1 out]
          }
          frame True {
          }
        }
      }
      event "密码锁": Value Change {
        n289 = event-data() -> ("NewVal"=w403:bool)  [unwired: 1 in, 5 out]
        n290 = case shown="假" w403 {
          frame False {
            n291 = local write "密码"(0.0 ("密码")) -> ()
          }
          frame True {
            n292 = call "数字键盘.vi"("显示样式"=u32 2) -> ("NewNumber"=→"密码":dbl)  [unwired: 1 in]
          }
        }
      }
      event "周期设置": Mouse Down {
        n293 = event-data() -> ()  [unwired: 1 in, 6 out]
        n294 = global read "断电保存变量.vi" "定时控制输入"() -> (w408:T11)
        n295 = call "周期设置.vi"("定时控制输入"=w408) -> ("定时控制输出"=w407:T11)  [unwired: 10 in]
        n296 = global write "断电保存变量.vi" "定时控制输入"(w407) -> ()
      }
      event "水样测试": Value Change {
        n297 = event-data() -> ()  [unwired: 1 in, 6 out]
        n298 = call "水样测试配置.vi"() -> ("确认输出"=w410:bool, "水样测定时间输出"=w409:dbl)  [unwired: 10 in]
        n299 = case shown="真" w410 {
          tunnel: w409 -> [_ w413]
          frame False {
          }
          frame True {
            n300 = vi-ref "水样测试.vi"() -> (w414:refnum<vi>)
            n301 = property class="VI"(reference=w414) -> ("Name"=w418:string, "Exec.State"=w416:T12)  [unwired: 1 in, 2 out]
            n302 = Open VI Reference(type specifier VI Refnum (for type only)=refnum<vi> refnum, vi path=w418, options=128 ("选项")) -> (vi reference=w419:refnum<vi>)  [unwired: 3 in, 1 out]
            n303 = case shown="\"Idle\"" w416 {
              tunnel: [w420 w424] -> w415
              tunnel: w419 -> [w420 w423]
              tunnel: w413 -> [_ w422]
              tunnel: "hd" ("数据标记表") -> [_ w421]
              frame "Bad", Default {
              }
              frame "Idle" {
                n304 = call-by-ref "开始异步调用"(reference=w423, "数据标记表"=w421, "水样测试时间"=w422) -> (reference out=w424:refnum<vi>)  [unwired: 11 in, 1 out]
              }
            }
            n305 = Close Reference(reference=w415) -> ()  [unwired: 1 in, 1 out]
          }
        }
      }
      event "标样核查": Value Change {
        n306 = event-data() -> ()  [unwired: 1 in, 6 out]
        n307 = call "标样核查配置.vi"() -> ("确认输出"=w426:bool, "标样核查配置"=w425:T15)  [unwired: 10 in]
        n308 = case shown="真" w426 {
          tunnel: w425 -> [_ w427]
          frame False {
          }
          frame True {
            n309 = vi-ref "标样核查.vi"() -> (w428:refnum<vi>)
            n310 = property class="VI"(reference=w428) -> ("Name"=w433:string, "Exec.State"=w430:T12)  [unwired: 1 in, 2 out]
            n311 = Open VI Reference(type specifier VI Refnum (for type only)=refnum<vi> refnum, vi path=w433, options=128 ("选项")) -> (vi reference=w434:refnum<vi>)  [unwired: 3 in, 1 out]
            n312 = case shown="\"Idle\"" w430 {
              tunnel: [w435 w438] -> w429
              tunnel: w434 -> [w435 w437]
              tunnel: w427 -> [_ w436]
              frame "Bad", Default {
              }
              frame "Idle" {
                n313 = call-by-ref "开始异步调用"(reference=w437, "标样核查配置"=w436) -> (reference out=w438:refnum<vi>)  [unwired: 12 in, 1 out]
              }
            }
            n314 = Close Reference(reference=w429) -> ()  [unwired: 1 in, 1 out]
          }
        }
      }
      event "停止": Value Change {
        n315 = event-data() -> ()  [unwired: 1 in, 6 out]
        n316 = Send Notification(notification=TRUE ("通知"), notifier=w440) -> ()  [unwired: 1 in, 2 out]
      }
      event "open MB": Value Change {
        n317 = event-data() -> ()  [unwired: 1 in, 6 out]
        n318 = Flush Queue(queue=w443) -> (queue out=w442:refnum<queue>)  [unwired: 1 in, 2 out]
        n319 = Enqueue Element(queue=w442, element="open" ("元素")) -> ()  [unwired: 2 in, 3 out]
      }
      event "设置": Value Change {
        n320 = event-data() -> ()  [unwired: 1 in, 6 out]
        n321 = property on="窗格" class="Pane"("Origin"=T2 {"Horizontal"=0, "Vertical"=628} ("原点")) -> ()  [unwired: 2 in, 2 out]
      }
      event "pH", "DO", "Turb", "Cond", "Temp", "叶绿素a启用", "蓝绿藻", "pH探头选择", "DO探头选择", "电导率探头选择", "浊度探头选择", "叶绿素a探头选择", "蓝绿藻探头选择", "VISA资源名称": Value Change {
        n322 = event-data() -> ()  [unwired: 1 in, 6 out]
        n323 = flat-sequence {
          frame #0 {
            n324 = global write "断电保存变量.vi" "Cond"("Cond") -> ()
            n325 = global write "断电保存变量.vi" "Temp"("Temp") -> ()
            n326 = global write "断电保存变量.vi" "DO"("DO") -> ()
            n327 = global write "断电保存变量.vi" "Turb"("Turb") -> ()
            n328 = global write "断电保存变量.vi" "pH"("pH") -> ()
            n329 = global write "断电保存变量.vi" "蓝绿藻"("蓝绿藻") -> ()
            n330 = global write "断电保存变量.vi" "叶绿素a启用"("叶绿素a启用") -> ()
            n331 = global write "断电保存变量.vi" "VISA资源名称"("VISA资源名称") -> ()
            n332 = global read "断电保存变量.vi" "探头选择"() -> (w452:T3)
            n333 = Bundle By Name(cluster=w452, "pH探头选择"="pH探头选择", "DO探头选择"="DO探头选择", "电导率探头选择"="电导率探头选择", "浊度探头选择"="浊度探头选择", "叶绿素a探头选择"="叶绿素a探头选择", "蓝绿藻探头选择"="蓝绿藻探头选择") -> (w451:T3)
            n334 = global write "断电保存变量.vi" "探头选择"(w451) -> ()
          }
          frame #1 {
            n335 = call <vilib>:"Application Directory.vi"() -> ("Application Directory"=w470:path)
            n336 = Build Path(base path=w470, name or relative path="data\\set.ini" ("名称或相对路径")) -> (appended path=w469:path)
            n337 = call <vilib>:"Open Config Data.vi"("configuration file path"=w469) -> ("error out"=w473:errorcluster, "refnum"=w474:T14)  [unwired: 8 in, 1 out]
            n338 = vi-ref "断电保存变量.vi"() -> (w467:refnum<vi>)
            n339 = call <userlib>:"Write Panel to INI__ogtk.vi"("error in (no error)"=w473, "VI ref"=w467, "refnum"=w474) -> ("error out"=w471:errorcluster, "refnum out"=w472:T14)  [unwired: 7 in]
            n340 = call <vilib>:"Close Config Data.vi"("error in (no error)"=w471, "refnum"=w472) -> ("error out"=w463:errorcluster, "file path"=w464:path)  [unwired: 8 in]
            n341 = Open/Create/Replace File(file path (use dialog)=w464, error in=w463) -> (refnum out=w465:refnum<file>, error out=w466:errorcluster)  [unwired: 4 in, 1 out]
            n342 = Flush File(refnum=w465, error in=w466) -> (refnum out=w461:refnum<file>, error out=w462:errorcluster)
            n343 = Close File(refnum=w461, error in=w462) -> ()  [unwired: 2 out]
          }
          frame #2 {
          }
        }
      }
      event "打开串口": Value Change {
        n344 = event-data() -> ()  [unwired: 1 in, 6 out]
        n345 = global read "多参数全局变量.vi" "MB_Serial session"() -> (w480:refnum<class "MB_Master_Serial.lvclass">)
        n346 = property class="MB_Master_Serial"(reference=w480) -> ("Properties:Session Valid"=w479:bool)  [unwired: 1 in, 2 out]
        n347 = Select(t="close" ("元素"), s=w479, f="open" ("元素")) -> (s? t:f=w476:string)
        n348 = Enqueue Element(queue=w475, element=w476) -> ()  [unwired: 2 in, 3 out]
      }
      event "探头校正返回", "设置页返回": Value Change {
        n349 = event-data() -> ()  [unwired: 1 in, 6 out]
        n350 = property on="窗格" class="Pane"("Origin"=T2 {"Horizontal"=0, "Vertical"=0} ("原点")) -> ()  [unwired: 2 in, 2 out]
      }
      event "探头校正", "水温校准": Value Change {
        n351 = event-data() -> ()  [unwired: 1 in, 6 out]
        n352 = vi-ref "水温校准.vi"() -> (w482:refnum<vi>)
        n353 = property on="窗格" class="Pane"("Origin"=T2 {"Horizontal"=1656, "Vertical"=0} ("原点")) -> ()  [unwired: 2 in, 2 out]
        n354 = property class="VI"(reference=w482) -> (reference out=w484:refnum<vi>, "Exec.State"=w483:T12)  [unwired: 1 in, 1 out]
        n355 = case shown="\"Bad\", 默认" w483 {
          tunnel: [w488 w490] -> w486
          tunnel: w484 -> [w488 w489]
          frame "Bad", Default {
          }
          frame "Idle" {
            n356 = invoke class="VI" method="Run VI"(reference=w489, "Wait until done"=FALSE ("结束前等待"), "Auto Dispose Ref"=FALSE ("自动销毁引用")) -> (reference out=w490:refnum<vi>)  [unwired: 2 in, 4 out]
          }
        }
        n357 = invoke on="探头校准子面板" class="SubPnl" method="Remove VI"() -> (error out=w485:errorcluster)  [unwired: 3 in, 2 out]
        n358 = invoke on="探头校准子面板" class="SubPnl" method="Insert VI"(error in=w485, "VI Ref"=w486) -> ()  [unwired: 2 in, 4 out]
      }
      event "pH校准": Value Change {
        n359 = event-data() -> ()  [unwired: 1 in, 6 out]
        n360 = global read "断电保存变量.vi" "探头选择"() -> (w495:T3)
        n361 = Unbundle By Name(w495) -> ("pH探头选择"=w494:u16)
        n362 = case shown="1" w494 {
          tunnel: [w500 w501] -> w493
          frame 0, Default {
            n363 = vi-ref "斯坦道多参数.lvlib:禹山pH校准.vi"() -> (w500:refnum<vi>)
          }
          frame 1 {
            n364 = vi-ref "斯坦道多参数.lvlib:pH电极校准.vi"() -> (w501:refnum<vi>)
          }
        }
        n365 = property class="VI"(reference=w493) -> (reference out=w497:refnum<vi>, "Exec.State"=w496:T12)  [unwired: 1 in, 1 out]
        n366 = case shown="\"Bad\", 默认" w496 {
          tunnel: w497 -> [w502 w506]
          tunnel: [w502 w503] -> w499
          frame "Bad", Default {
          }
          frame "Idle" {
            n367 = invoke class="VI" method="Run VI"(reference=w506, "Wait until done"=FALSE ("结束前等待"), "Auto Dispose Ref"=FALSE ("自动销毁引用")) -> (reference out=w503:refnum<vi>)  [unwired: 2 in, 4 out]
          }
        }
        n368 = invoke on="探头校准子面板" class="SubPnl" method="Remove VI"() -> (error out=w498:errorcluster)  [unwired: 3 in, 2 out]
        n369 = invoke on="探头校准子面板" class="SubPnl" method="Insert VI"(error in=w498, "VI Ref"=w499) -> ()  [unwired: 2 in, 4 out]
      }
      event "电导率校准": Value Change {
        n370 = event-data() -> ()  [unwired: 1 in, 6 out]
        n371 = global read "断电保存变量.vi" "探头选择"() -> (w509:T3)
        n372 = Unbundle By Name(w509) -> ("电导率探头选择"=w508:u16)
        n373 = case shown="0, 默认" w508 {
          tunnel: [w514 w515] -> w507
          frame 0, Default {
            n374 = vi-ref "斯坦道多参数.lvlib:禹山电导率校准.vi"() -> (w514:refnum<vi>)
          }
          frame 1 {
            n375 = vi-ref "斯坦道多参数.lvlib:电导率电极校准.vi"() -> (w515:refnum<vi>)
          }
        }
        n376 = property class="VI"(reference=w507) -> (reference out=w511:refnum<vi>, "Exec.State"=w510:T12)  [unwired: 1 in, 1 out]
        n377 = case shown="\"Bad\", 默认" w510 {
          tunnel: [w516 w518] -> w513
          tunnel: w511 -> [w516 w517]
          frame "Bad", Default {
          }
          frame "Idle" {
            n378 = invoke class="VI" method="Run VI"(reference=w517, "Wait until done"=FALSE ("结束前等待"), "Auto Dispose Ref"=FALSE ("自动销毁引用")) -> (reference out=w518:refnum<vi>)  [unwired: 2 in, 4 out]
          }
        }
        n379 = invoke on="探头校准子面板" class="SubPnl" method="Remove VI"() -> (error out=w512:errorcluster)  [unwired: 3 in, 2 out]
        n380 = invoke on="探头校准子面板" class="SubPnl" method="Insert VI"(error in=w512, "VI Ref"=w513) -> ()  [unwired: 2 in, 4 out]
      }
      event "溶解氧校准": Value Change {
        n381 = event-data() -> ()  [unwired: 1 in, 6 out]
        n382 = global read "断电保存变量.vi" "探头选择"() -> (w523:T3)
        n383 = Unbundle By Name(w523) -> ("DO探头选择"=w522:u16)
        n384 = case shown="1" w522 {
          tunnel: [w528 w529] -> w521
          frame 0, Default {
            n385 = vi-ref "斯坦道多参数.lvlib:禹山溶解氧校准.vi"() -> (w528:refnum<vi>)
          }
          frame 1 {
            n386 = vi-ref "斯坦道多参数.lvlib:溶解氧电极校准.vi"() -> (w529:refnum<vi>)
          }
        }
        n387 = property class="VI"(reference=w521) -> (reference out=w525:refnum<vi>, "Exec.State"=w524:T12)  [unwired: 1 in, 1 out]
        n388 = case shown="\"Bad\", 默认" w524 {
          tunnel: [w530 w532] -> w527
          tunnel: w525 -> [w530 w531]
          frame "Bad", Default {
          }
          frame "Idle" {
            n389 = invoke class="VI" method="Run VI"(reference=w531, "Wait until done"=FALSE ("结束前等待"), "Auto Dispose Ref"=FALSE ("自动销毁引用")) -> (reference out=w532:refnum<vi>)  [unwired: 2 in, 4 out]
          }
        }
        n390 = invoke on="探头校准子面板" class="SubPnl" method="Remove VI"() -> (error out=w526:errorcluster)  [unwired: 3 in, 2 out]
        n391 = invoke on="探头校准子面板" class="SubPnl" method="Insert VI"(error in=w526, "VI Ref"=w527) -> ()  [unwired: 2 in, 4 out]
      }
      event "浊度校准": Value Change {
        n392 = event-data() -> ()  [unwired: 1 in, 6 out]
        n393 = global read "断电保存变量.vi" "探头选择"() -> (w537:T3)
        n394 = Unbundle By Name(w537) -> ("浊度探头选择"=w536:u16)
        n395 = case shown="1" w536 {
          tunnel: [w542 w543] -> w535
          frame 0, Default {
            n396 = vi-ref "斯坦道多参数.lvlib:禹山浊度校准.vi"() -> (w542:refnum<vi>)
          }
          frame 1 {
            n397 = vi-ref "斯坦道多参数.lvlib:浊度电极校准.vi"() -> (w543:refnum<vi>)
          }
        }
        n398 = property class="VI"(reference=w535) -> (reference out=w539:refnum<vi>, "Exec.State"=w538:T12)  [unwired: 1 in, 1 out]
        n399 = case shown="\"Bad\", 默认" w538 {
          tunnel: [w544 w546] -> w541
          tunnel: w539 -> [w544 w545]
          frame "Bad", Default {
          }
          frame "Idle" {
            n400 = invoke class="VI" method="Run VI"(reference=w545, "Wait until done"=FALSE ("结束前等待"), "Auto Dispose Ref"=FALSE ("自动销毁引用")) -> (reference out=w546:refnum<vi>)  [unwired: 2 in, 4 out]
          }
        }
        n401 = invoke on="探头校准子面板" class="SubPnl" method="Remove VI"() -> (error out=w540:errorcluster)  [unwired: 3 in, 2 out]
        n402 = invoke on="探头校准子面板" class="SubPnl" method="Insert VI"(error in=w540, "VI Ref"=w541) -> ()  [unwired: 2 in, 4 out]
      }
      event "叶绿素a校准": Value Change {
        n403 = event-data() -> ()  [unwired: 1 in, 6 out]
        n404 = vi-ref "禹山叶绿素a校准.vi"() -> (w549:refnum<vi>)
        n405 = property class="VI"(reference=w549) -> (reference out=w551:refnum<vi>, "Exec.State"=w550:T12)  [unwired: 1 in, 1 out]
        n406 = case shown="\"Bad\", 默认" w550 {
          tunnel: [w554 w556] -> w553
          tunnel: w551 -> [w554 w555]
          frame "Bad", Default {
          }
          frame "Idle" {
            n407 = invoke class="VI" method="Run VI"(reference=w555, "Wait until done"=FALSE ("结束前等待"), "Auto Dispose Ref"=FALSE ("自动销毁引用")) -> (reference out=w556:refnum<vi>)  [unwired: 2 in, 4 out]
          }
        }
        n408 = invoke on="探头校准子面板" class="SubPnl" method="Remove VI"() -> (error out=w552:errorcluster)  [unwired: 3 in, 2 out]
        n409 = invoke on="探头校准子面板" class="SubPnl" method="Insert VI"(error in=w552, "VI Ref"=w553) -> ()  [unwired: 2 in, 4 out]
      }
    }
  }
  n410 = while {
    tunnel: w7 -> [w560]
    stop <- FALSE stop-if-true
    n411 = Dequeue Element(queue=w560) -> (element=w559:string)  [unwired: 2 in, 3 out]
    n412 = case shown="\"open\"" w559 {
      tunnel: [_ w564 w569] -> _
      frame "假", Default {
      }
      frame "open" {
        n413 = global read "多参数全局变量.vi" "MB_Serial session"() -> (w563:refnum<class "MB_Master_Serial.lvclass">)
        n414 = global read "断电保存变量.vi" "VISA资源名称"() -> (w566:refnum<visa-resource-name>)
        n415 = call "close MB.vi"("MB_Serial session"=w563) -> ("error out"=w567:errorcluster)  [unwired: 10 in]
        n416 = call "open MB.vi"("error in (no error)"=w567, "Serial Config"=T16 {"baud rate (bps)"=9600, "stop bits"=10, "parity"=0, "flow control"=0, "timeout"=1000, "retries"=1}, "VISA资源名称"=w566) -> ("error out"=w564:errorcluster, "MB_Serial session"=w562:refnum<class "MB_Master_Serial.lvclass">)  [unwired: 7 in]
        n417 = global write "多参数全局变量.vi" "MB_Serial session"(w562) -> ()
      }
      frame "close" {
        n418 = global read "多参数全局变量.vi" "MB_Serial session"() -> (w568:refnum<class "MB_Master_Serial.lvclass">)
        n419 = call "close MB.vi"("MB_Serial session"=w568) -> ("error out"=w569:errorcluster)  [unwired: 10 in]
      }
    }
  }
